vi "AvancerGyro.vi"(10 "Ajustement":dbl, 11 "Vitesse":dbl) -> ()   [LabVIEW 2016]
uses:
  <vilib>/Rock Robotics/WPI/Utilities/WPI_GetSetVariantRefNum.vi
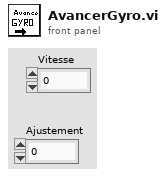
[diagram p1: front panel]
types:
  T1 = typedef "WPI_GyroDevRef.ctl" = cluster{"DevStatus":errorcluster, "Analog Channel":T2, "Offset":dbl, "Gain (VoltsPerDegree/Second)":dbl, "Gyro Type":enum16{"Analog", "XRS450"}, "Handle":i32, "SPI Bus":T3, "Device Found":bool, "Sample Rate":dbl, "Calibrate On Open":bool}
  T2 = typedef "FPGA_AIChannel.ctl" = enum8{"AI 0", "AI 1", "AI 2", "AI 3", "AI MXP 0", "AI MXP 1", "AI MXP 2", "AI MXP 3", "Invalid"}
  T3 = typedef "spi_bus.ctl" = enum16{"SPI On-Board, CS0", "SPI On-Board, CS1", "SPI On-Board, CS2", "SPI On-Board, CS3", "SPI MXP", "Invalid"}
  T4 = typedef "WPI_RobotDriveDevRef.ctl" = cluster{"DevStatus":errorcluster, "Motors[]":T5[], "Square Inputs":bool, "Max Output":dbl}
  T5 = typedef "WPI_MotorControlDeviceRef.ctl" = cluster{"DeviceStatus":errorcluster, "Type":T6, "PWM":cluster{"PWM Channel":T7, "DeadBand":T8}, "CAN":cluster{"Device Number":u8, "SetOutput VI Ref":variant, "GetOutput VI Ref":variant, "Enable VI Ref":variant, "Disable VI Ref":variant, "Data":variant}, "Invert":bool}
  T6 = typedef "WPI_MotorControlType.ctl" = enum16{"PWM", "CAN"}
  T7 = typedef "FPGA_DIOPWMChannel.ctl" = enum8{"PWM 0", "PWM 1", "PWM 2", "PWM 3", "PWM 4", "PWM 5", "PWM 6", "PWM 7", "PWM 8", "PWM 9", "PWM MXP 0", "PWM MXP 1", "PWM MXP 2", "PWM MXP 3", "PWM MXP 4", "PWM MXP 5", "PWM MXP 6", "PWM MXP 7", "PWM MXP 8", "PWM MXP 9", "Invalid"}
  T8 = typedef "WPI_PWMDeadband.ctl" = cluster{"Name":string, "maxPositivePwm":i32, "minPositivePwm":i32, "centerPwm":i32, "maxNegativePwm":i32, "minNegativePwm":i32, "angularRange":u16}
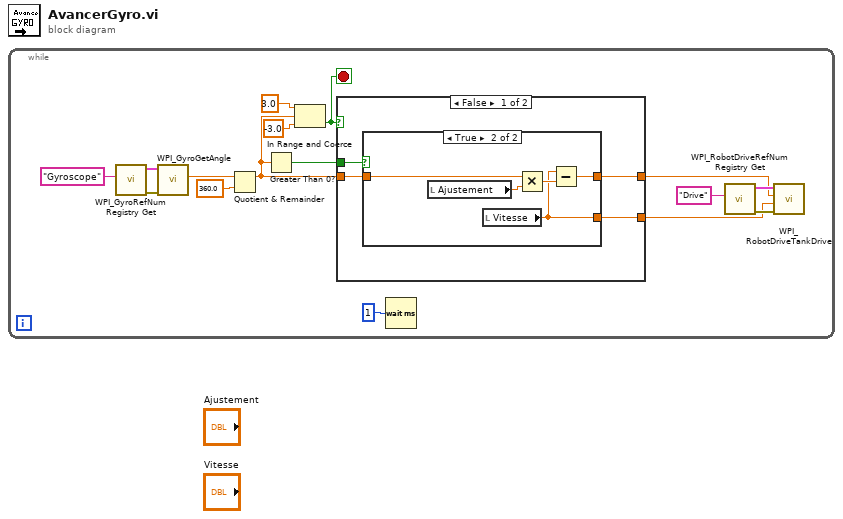
[diagram p0: block diagram]
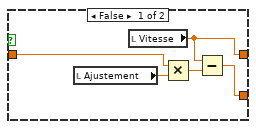
[diagram p2: hidden frame]
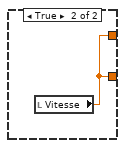
[diagram p3: hidden frame]
diagram:
  n1 = while {
    stop <- w5 stop-if-true
    n2 = call <vilib>:"WPI_GyroRefNum Registry Get.vi"("refnum name"="Gyroscope") -> ("error out"=w14:errorcluster, "GyroDevRef"=w15:T1)  [unwired: 9 in]
    n3 = call <vilib>:"WPI_GyroGetAngle.vi"("error in"=w14, "GyroDevRef"=w15) -> ("Angle"=w3:dbl)  [unwired: 5 in, 4 out]
    n4 = Quotient & Remainder(x=w3, y=360.0) -> (x-y*floor(x/y)=w1:dbl)  [unwired: 1 out]
    n5 = Greater Than 0?(x=w1) -> (x > 0?=w11:bool)
    n6 = In Range and Coerce(upper limit=3.0, x=w1, lower limit=-3.0) -> (In Range?=w5:bool)  [unwired: 1 out]
    n7 = case shown="False" w5 {
      tunnel: w11 -> [w20 _]
      tunnel: [w18 w31] -> w7
      tunnel: [w19 w31] -> w6
      tunnel: w1 -> [w17 _]
      frame False {
        n8 = case shown="True" w20 {
          tunnel: [w24 w28] -> w19
          tunnel: [w23 w29] -> w18
          tunnel: w17 -> [w21 w27]
          frame False {
            n9 = local read "Ajustement"() -> (w22:dbl)
            n10 = local read "Vitesse"() -> (w23:dbl)
            n11 = Multiply(x=w21, y=w22) -> (x*y=w25:dbl)
            n12 = Subtract(x=w23, y=w25) -> (x-y=w24:dbl)
          }
          frame True {
            n13 = local read "Ajustement"() -> (w26:dbl)
            n14 = local read "Vitesse"() -> (w28:dbl)
            n15 = Multiply(x=w27, y=w26) -> (x*y=w30:dbl)
            n16 = Subtract(x=w28, y=w30) -> (x-y=w29:dbl)
          }
        }
      }
      frame True {
        n17 = local read "Vitesse"() -> (w31:dbl)
      }
    }
    n18 = Wait (ms)(milliseconds to wait=u32 1) -> ()  [unwired: 1 out]
    n19 = call <vilib>:"WPI_RobotDriveRefNum Registry Get.vi"("refnum name"="Drive") -> ("error out"=w10:errorcluster, "RobotDriveDevRef"=w9:T4)  [unwired: 9 in]
    n20 = call <vilib>:"WPI_RobotDriveTankDrive.vi"("error in (no error)"=w10, "Right axis value"=w6, "Left axis value"=w7, "RobotDriveDevRef"=w9) -> ()  [unwired: 5 in, 3 out]
  }
